vi "test_MonoInit.vi"(8 "error in":errorcluster, 10 "force":bool=TRUE, 11 "Monochromator in":refnum<class "Monochromator.lvclass">) -> (0 "error out":errorcluster, 2 "iterations":i32, 3 "Monochromator out":refnum<class "Monochromator.lvclass">)   [LabVIEW 2020, in "horiba.test.lvlib"]
uses:
  horiba.test.lvlib
  Classes/Mono/Monochromator.lvclass
  <vilib>/addons/_JKI Toolkits/Caraya/classes/Assert/Assert True.vi
panel:
  # "Connector Pane"
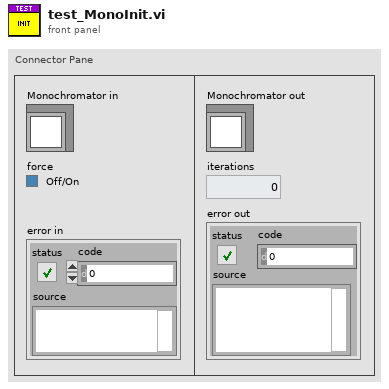
[diagram p1: front panel]
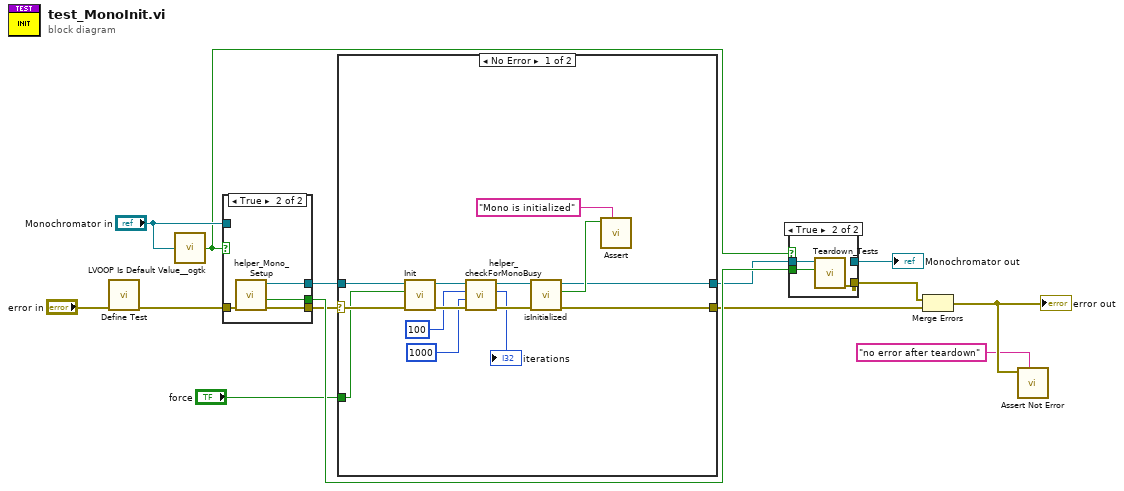
[diagram p0: block diagram]
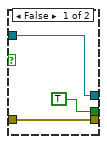
[diagram p2: hidden frame]
diagram:
  n1 = call <vilib>:"Define Test.vi"("error in (no error)"="error in") -> ("error out"=w8:errorcluster)  [unwired: 9 in, 1 out]
  n2 = call <userlib>:"LVOOP Is Default Value__ogtk.vi"("Object"="Monochromator in") -> ("Is Default Value?"=w9:bool)
  n3 = case shown="True" w9 {
    tunnel: w8 -> [w16 w21]
    tunnel: [w16 w20] -> w3
    tunnel: [w17 w19] -> w6
    tunnel: [TRUE ("Module Was Already Running?") w18] -> w11
    tunnel: "Monochromator in" -> [w17 _]
    frame False {
    }
    frame True {
      n4 = call "helper_Mono_Setup.vi"("error in"=w21) -> ("error out"=w20:errorcluster, "Module Was Already Running?"=w18:bool, "Monochromator out"=w19:refnum<class "Monochromator.lvclass">)  [unwired: 7 in, 1 out]
    }
  }
  n5 = case shown="No Error" w3 {
    selector: w3 -> [w33 w37]
    tunnel: [w25 w36] -> w5
    tunnel: w6 -> [w34 w36]
    tunnel: [w24 w37] -> w2
    tunnel: "force" -> [w22 _]
    frame No Error {
      n6 = call "Init.vi"("error in (no error)"=w33, "force"=w22, "Monochromator in"=w34) -> ("error out"=w32:errorcluster, "Monochromator out"=w31:refnum<class "Monochromator.lvclass">)  [unwired: 5 in, 2 out]
      n7 = call "helper_checkForMonoBusy.vi"("error in (no error)"=w32, "milliseconds to wait"=u32 1000, "Numeric"=100, "Monochromator in"=w31) -> ("error out"=w27:errorcluster, "iterations"=→"iterations":i32, "Monochromator out"=w28:refnum<class "Monochromator.lvclass">)  [unwired: 5 in]
      n8 = call "isInitialized.vi"("error in (no error)"=w27, "Monochromator in"=w28) -> ("error out"=w24:errorcluster, "mono is initialized?"=w26:bool, "Monochromator out"=w25:refnum<class "Monochromator.lvclass">)  [unwired: 7 in]
      n9 = call-poly <vilib>:"Assert.vi"("Label"="Mono is initialized", "True?"=w26) -> ()  [unwired: 8 in, 2 out]
    }
    frame Error {
    }
  }
  n10 = case shown="True" w9 {
    tunnel: w5 -> [w38 w41]
    tunnel: [_ w40] -> w7
    tunnel: w11 -> [_ w39]
    tunnel: [w38 _] -> w4
    frame False {
    }
    frame True {
      n11 = call "Teardown_Tests.vi"("Module Was Already Running?"=w39, "horiba.lvlib:GenericDevice"=w41) -> ("error out"=w40:errorcluster)  [unwired: 8 in, 1 out]
    }
  }
  "Monochromator out" <- w4
  n12 = Merge Errors(w7, w2) -> (w13:errorcluster)
  "error out" <- w13
  n13 = call <vilib>:"Assert Not Error.vi"("Label"="no error after teardown", "Not Error?"=w13) -> ()  [unwired: 8 in, 2 out]
